vi "Editing VI Descriptions-2015.vi"() -> ()   [LabVIEW 2015]
doc: "Created IvanLis by LabVIEW Portal\nProfile: http://labviewportal.org/memberlist.php?mode=viewprofile&u=987\neMail: IvanLisanov@gMail.com\nTelegram: https://t.me/IvanLis"
panel:
  out "File Select":i32
  out "File Number":i32
  in  "DeSelect File":bool
  in  "DeSelect":bool
  in  "Select":bool
  in  "Change Description":bool
  in  "Get File List":bool
  out "Update":bool
  in  "File Type":T1(ring)
  in  "Folder Select":path
  in  "Description":string="Created IvanLis by LabVIEW Portal\nProfile: http://labviewportal.org/memberlist.php?mode=viewprofile&u=987\neMail: IvanLisanov@gMail.com\nTelegram: https://t.me/IvanLis"
  in  "Array of File":cluster{"Change":bool, "File":string}[](array[cluster])
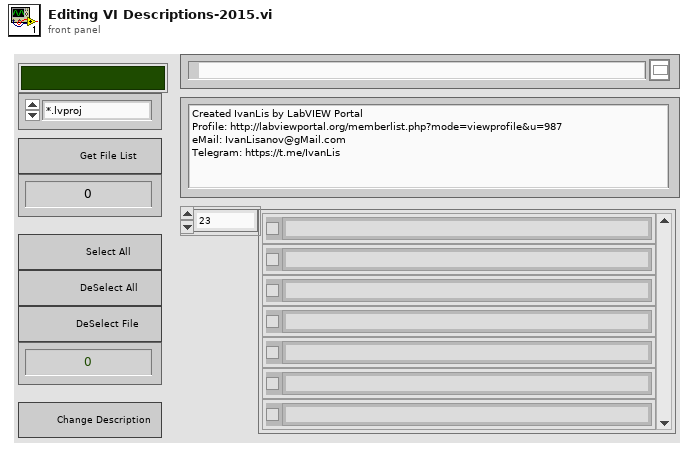
[diagram p1: front panel]
types:
  T1 = enum16{"*.lvproj", "*.vi", "*.ctl", "*.lvlib", "*.lvclass"}
  T2 = enum16{"open", "replace", "create", "open or create", "replace or create", "replace or create with confirmation"}
  T3 = typedef "LVRectTypeDef.ctl" = cluster{"Left":i16, "Top":i16, "Right":i16, "Bottom":i16}
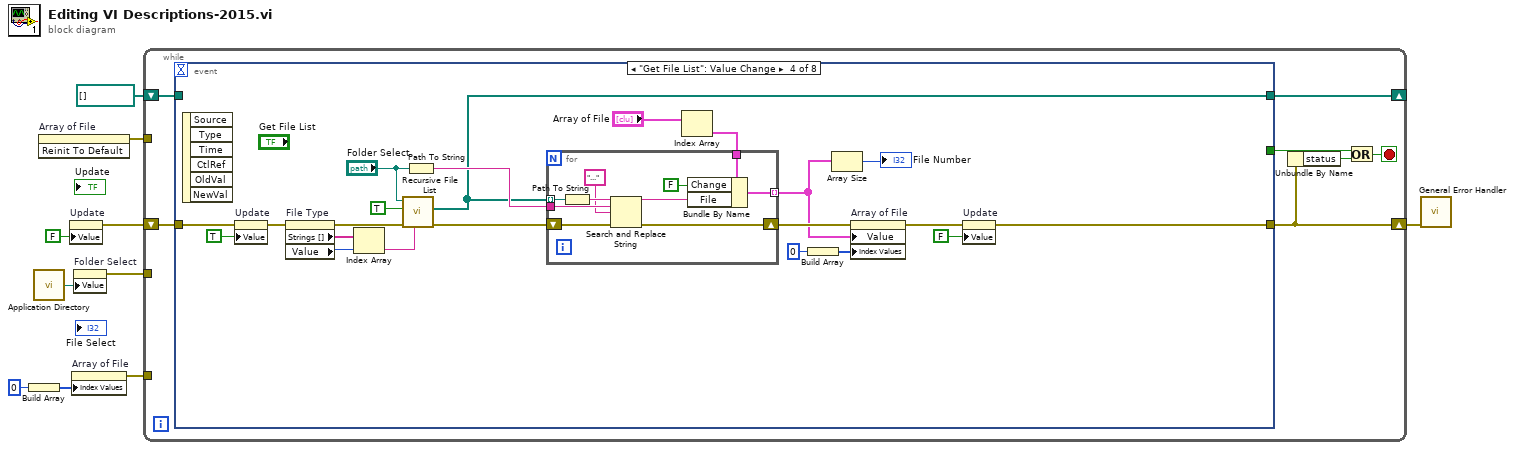
[diagram p0: block diagram]
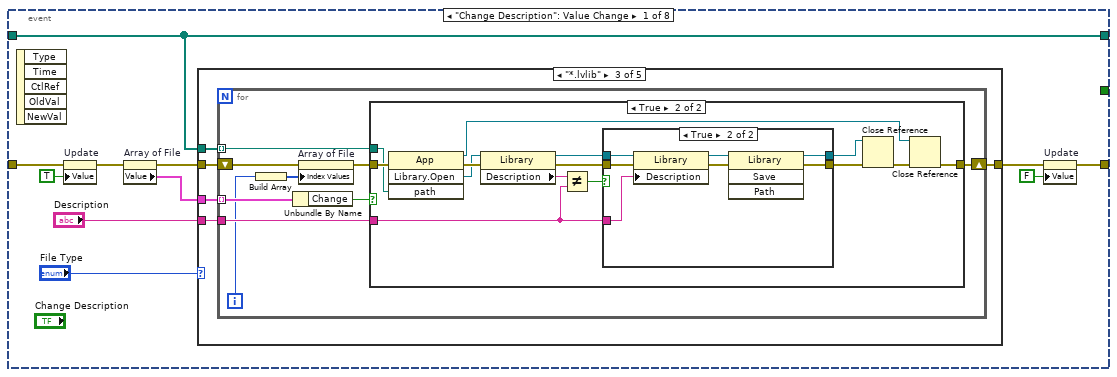
[diagram p2: hidden frame]
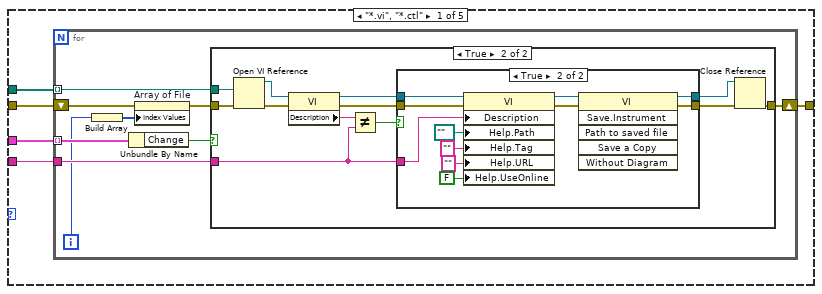
[diagram p3: hidden frame]
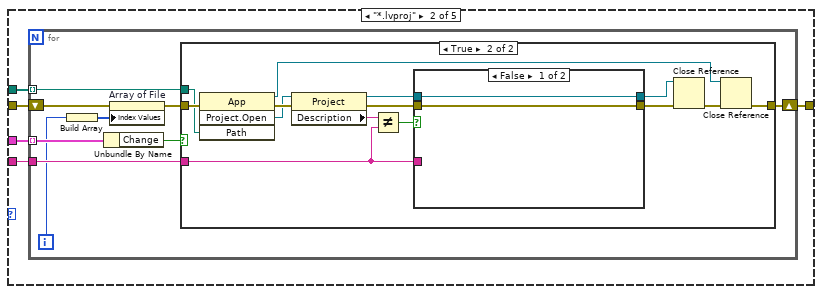
[diagram p6: hidden frame]
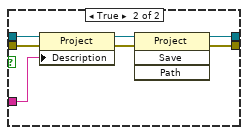
[diagram p8: hidden frame]
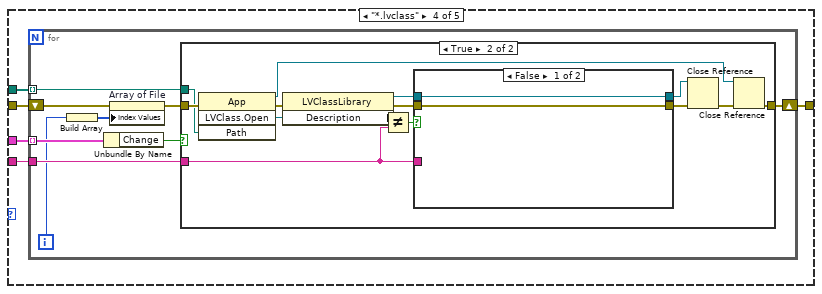
[diagram p11: hidden frame]
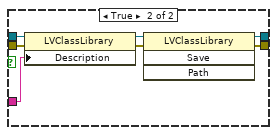
[diagram p13: hidden frame]
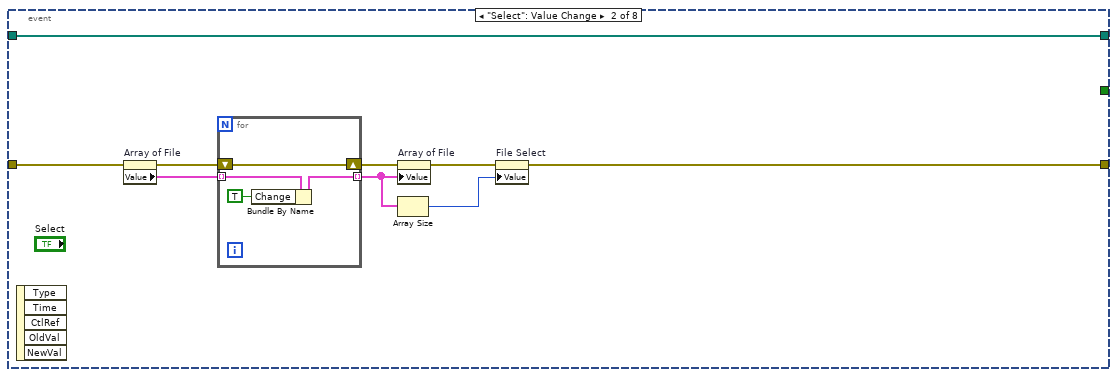
[diagram p15: hidden frame]
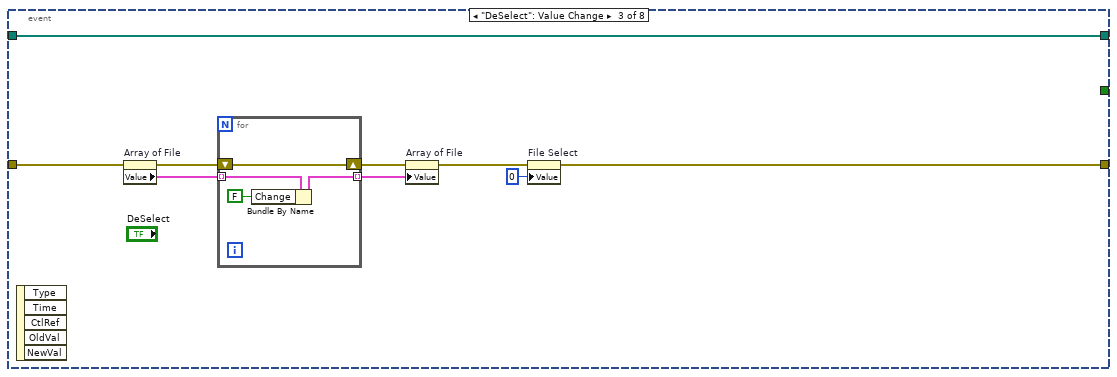
[diagram p16: hidden frame]
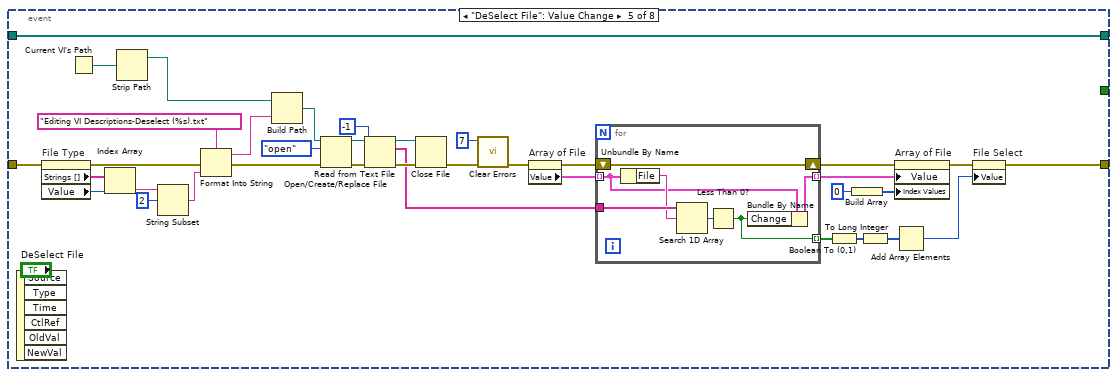
[diagram p17: hidden frame]
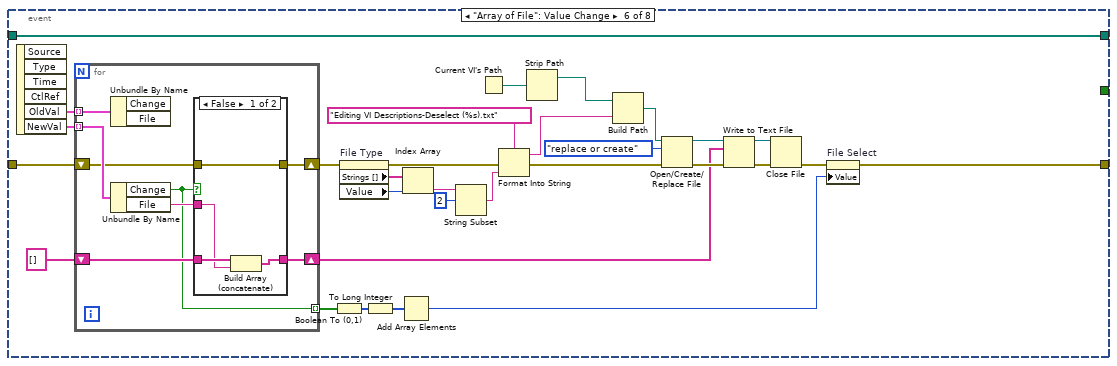
[diagram p18: hidden frame]
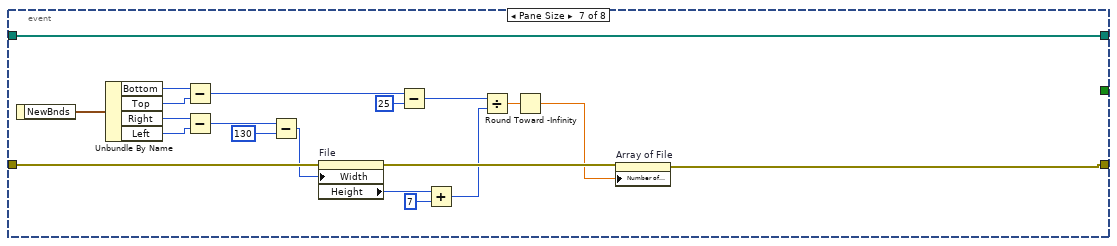
[diagram p20: hidden frame]
diagram:
  n1 = Build Array(u32 0) -> (w3:u32[])
  n2 = call <vilib>:"Application Directory.vi"() -> ("Application Directory"=w5:path)
  n3 = invoke on="Array of File" class="Arr (strict)" method="Reinit To Default"() -> (error out=w4:errorcluster)  [unwired: 3 in, 2 out]
  n4 = property on="Update" class="Bool (strict)"("Value"=FALSE ("Update")) -> (error out=w7:errorcluster)  [unwired: 2 in, 1 out]
  n5 = property on="Array of File" class="Arr (strict)"("Index Values"=w3) -> (error out=w1:errorcluster)  [unwired: 2 in, 1 out]
  n6 = property on="Folder Select" class="Path"("Value"=w5) -> (error out=w6:errorcluster)  [unwired: 2 in, 1 out]
  n7 = while {
    shift-right: [w16] -> w9
    shift-left: w7 -> [w17]
    shift-right: [w14] -> _
    shift-left: path[] [] ("All Files in Dir") -> [w13]
    tunnel: w6 -> [_]
    tunnel: w4 -> [_]
    tunnel: w1 -> [_]
    stop <- w15 stop-if-true
    n8 = event shown="[3] \"Get File List\": Value Change" {
      selector: _ -> [_ _ _ _ _ _ _ _]
      dyn-events: _ -> [_ _ _ _ _ _ _ _]
      timeout: _ -> [_ _ _ _ _ _ _ _]
      tunnel: w17 -> [w19 w192 w205 w213 w250 w312 w347 w351]
      tunnel: [w23 w186 w198 w220 w244 w289 w333 w351] -> w16
      tunnel: [w25 w189 w202 w224 w277 w311 w348 w350] -> w14
      tunnel: w13 -> [w25 w189 w202 _ w277 w311 w348 w350]
      tunnel: [_ _ _ _ _ _ _ w349] -> w12
      event "Change Description": Value Change {
        n9 = event-data() -> ()  [unwired: 1 in, 5 out]
        n10 = property on="Update" class="Bool (strict)"(error in=w19, "Value"=TRUE ("Update")) -> (error out=w20:errorcluster)  [unwired: 1 in, 1 out]
        n11 = property on="Array of File" class="Arr (strict)"(error in=w20) -> (error out=w27:errorcluster, "Value"=w26:cluster{"Change":bool, "File":string}[])  [unwired: 1 in, 1 out]
        n12 = case shown="\"*.lvlib\"" "File Type" {
          tunnel: "Description" -> [w33 w73 w111 w149 _]
          tunnel: w27 -> [w32 w72 w110 w148 w183]
          tunnel: w26 -> [w31 w71 w109 w147 _]
          tunnel: w25 -> [w30 w70 w108 w146 _]
          tunnel: [w29 w69 w107 w145 w183] -> w24
          frame "*.vi", "*.ctl" {
            n13 = for {
              tunnel: w33 -> [w41]
              shift-right: [w42] -> w29
              shift-left: w32 -> [w36]
              tunnel: w30 -> [w38] mode=indexing
              tunnel: w31 -> [w40] mode=indexing
              i -> [w34]
              n14 = Build Array(w34) -> (w37:i32[])
              n15 = Unbundle By Name(w40) -> ("Change"=w39:bool)
              n16 = property on="Array of File" class="Arr (strict)"(error in=w36, "Index Values"=w37) -> (error out=w35:errorcluster)  [unwired: 1 in, 1 out]
              n17 = case shown="True" w39 {
                tunnel: [w43 w55] -> w42
                tunnel: w41 -> [_ w46]
                tunnel: w35 -> [w43 w52]
                tunnel: w38 -> [_ w51]
                frame False {
                }
                frame True {
                  n18 = Open VI Reference(vi path=w51, error in (no error)=w52) -> (vi reference=w49:refnum<vi>, error out=w50:errorcluster)  [unwired: 4 in]
                  n19 = property class="VI"(reference=w49, error in=w50) -> (reference out=w48:refnum<vi>, error out=w44:errorcluster, "Description"=w47:string)
                  n20 = Not Equal?(x=w47, y=w46) -> (x != y?=w45:bool)
                  n21 = case shown="True" w45 {
                    tunnel: [w56 w66] -> w54
                    tunnel: [w57 w65] -> w53
                    tunnel: w48 -> [w57 w59]
                    tunnel: w46 -> [_ w58]
                    tunnel: w44 -> [w56 w60]
                    frame False {
                    }
                    frame True {
                      n22 = property class="VI"(reference=w59, error in=w60, "Description"=w58, "Help.Path"=path "" ("Help:Document Path"), "Help.Tag"="" ("Help:Document Tag"), "Help.URL"="" ("Help:Document Web URL"), "Help.UseOnline"=FALSE ("Help:Use Web URL")) -> (reference out=w67:refnum<vi>, error out=w68:errorcluster)
                      n23 = invoke class="VI" method="Save.Instrument"(reference=w67, error in=w68) -> (reference out=w65:refnum<vi>, error out=w66:errorcluster)  [unwired: 4 in, 4 out]
                    }
                  }
                  n24 = Close Reference(reference=w53, error in (no error)=w54) -> (error out=w55:errorcluster)
                }
              }
            }
          }
          frame "*.lvproj" {
            n25 = for {
              tunnel: w73 -> [w81]
              shift-right: [w82] -> w69
              shift-left: w72 -> [w76]
              tunnel: w70 -> [w78] mode=indexing
              tunnel: w71 -> [w80] mode=indexing
              i -> [w74]
              n26 = Build Array(w74) -> (w77:i32[])
              n27 = Unbundle By Name(w80) -> ("Change"=w79:bool)
              n28 = property on="Array of File" class="Arr (strict)"(error in=w76, "Index Values"=w77) -> (error out=w75:errorcluster)  [unwired: 1 in, 1 out]
              n29 = case shown="True" w79 {
                tunnel: [w83 w86] -> w82
                tunnel: w81 -> [_ w91]
                tunnel: w75 -> [w83 w95]
                tunnel: w78 -> [_ w87]
                frame False {
                }
                frame True {
                  n30 = invoke class="App" method="Project.Open"(error in=w95, "Path"=w87) -> (reference out=w84:refnum<vi>, error out=w94:errorcluster, "Project:Open"=w88:refnum<vi>)  [unwired: 2 in, 1 out]
                  n31 = property class="Project"(reference=w88, error in=w94) -> (reference out=w93:refnum<vi>, error out=w89:errorcluster, "Description"=w92:string)
                  n32 = Not Equal?(x=w92, y=w91) -> (x != y?=w90:bool)
                  n33 = case shown="False" w90 {
                    tunnel: [w98 w104] -> w97
                    tunnel: [w99 w103] -> w96
                    tunnel: w93 -> [w99 w101]
                    tunnel: w91 -> [_ w100]
                    tunnel: w89 -> [w98 w102]
                    frame False {
                    }
                    frame True {
                      n34 = property class="Project"(reference=w101, error in=w102, "Description"=w100) -> (reference out=w105:refnum<vi>, error out=w106:errorcluster)
                      n35 = invoke class="Project" method="Save"(reference=w105, error in=w106) -> (reference out=w103:refnum<vi>, error out=w104:errorcluster)  [unwired: 2 in, 2 out]
                    }
                  }
                  n36 = Close Reference(reference=w96, error in (no error)=w97) -> (error out=w85:errorcluster)
                  n37 = Close Reference(reference=w84, error in (no error)=w85) -> (error out=w86:errorcluster)
                }
              }
            }
          }
          frame "*.lvlib" {
            n38 = for {
              tunnel: w111 -> [w119]
              shift-right: [w120] -> w107
              shift-left: w110 -> [w114]
              tunnel: w108 -> [w116] mode=indexing
              tunnel: w109 -> [w118] mode=indexing
              i -> [w112]
              n39 = Build Array(w112) -> (w115:i32[])
              n40 = Unbundle By Name(w118) -> ("Change"=w117:bool)
              n41 = property on="Array of File" class="Arr (strict)"(error in=w114, "Index Values"=w115) -> (error out=w113:errorcluster)  [unwired: 1 in, 1 out]
              n42 = case shown="True" w117 {
                tunnel: [w121 w124] -> w120
                tunnel: w119 -> [_ w129]
                tunnel: w113 -> [w121 w133]
                tunnel: w116 -> [_ w125]
                frame False {
                }
                frame True {
                  n43 = invoke class="App" method="Library.Open"(error in=w133, "path"=w125) -> (reference out=w122:refnum<vi>, error out=w132:errorcluster, "Open Library"=w126:refnum<vi>)  [unwired: 2 in, 1 out]
                  n44 = property class="Library"(reference=w126, error in=w132) -> (reference out=w131:refnum<vi>, error out=w127:errorcluster, "Description"=w130:string)
                  n45 = Not Equal?(x=w130, y=w129) -> (x != y?=w128:bool)
                  n46 = case shown="True" w128 {
                    tunnel: [w136 w142] -> w135
                    tunnel: [w137 w141] -> w134
                    tunnel: w131 -> [w137 w139]
                    tunnel: w129 -> [_ w138]
                    tunnel: w127 -> [w136 w140]
                    frame False {
                    }
                    frame True {
                      n47 = property class="Library"(reference=w139, error in=w140, "Description"=w138) -> (reference out=w143:refnum<vi>, error out=w144:errorcluster)
                      n48 = invoke class="Library" method="Save"(reference=w143, error in=w144) -> (reference out=w141:refnum<vi>, error out=w142:errorcluster)  [unwired: 2 in, 2 out]
                    }
                  }
                  n49 = Close Reference(reference=w134, error in (no error)=w135) -> (error out=w123:errorcluster)
                  n50 = Close Reference(reference=w122, error in (no error)=w123) -> (error out=w124:errorcluster)
                }
              }
            }
          }
          frame "*.lvclass" {
            n51 = for {
              tunnel: w149 -> [w157]
              shift-right: [w158] -> w145
              shift-left: w148 -> [w152]
              tunnel: w146 -> [w154] mode=indexing
              tunnel: w147 -> [w156] mode=indexing
              i -> [w150]
              n52 = Build Array(w150) -> (w153:i32[])
              n53 = Unbundle By Name(w156) -> ("Change"=w155:bool)
              n54 = property on="Array of File" class="Arr (strict)"(error in=w152, "Index Values"=w153) -> (error out=w151:errorcluster)  [unwired: 1 in, 1 out]
              n55 = case shown="True" w155 {
                tunnel: [w159 w162] -> w158
                tunnel: w157 -> [_ w167]
                tunnel: w151 -> [w159 w171]
                tunnel: w154 -> [_ w163]
                frame False {
                }
                frame True {
                  n56 = invoke class="App" method="LVClass.Open"(error in=w171, "Path"=w163) -> (reference out=w160:refnum<vi>, error out=w170:errorcluster, "LVClass.Open"=w164:refnum<vi>)  [unwired: 2 in, 1 out]
                  n57 = property class="LVClassLibrary"(reference=w164, error in=w170) -> (reference out=w169:refnum<vi>, error out=w165:errorcluster, "Description"=w168:string)
                  n58 = Not Equal?(x=w168, y=w167) -> (x != y?=w166:bool)
                  n59 = case shown="False" w166 {
                    tunnel: [w174 w180] -> w173
                    tunnel: [w175 w179] -> w172
                    tunnel: w169 -> [w175 w177]
                    tunnel: w167 -> [_ w176]
                    tunnel: w165 -> [w174 w178]
                    frame False {
                    }
                    frame True {
                      n60 = property class="LVClassLibrary"(reference=w177, error in=w178, "Description"=w176) -> (reference out=w181:refnum<vi>, error out=w182:errorcluster)
                      n61 = invoke class="LVClassLibrary" method="Save"(reference=w181, error in=w182) -> (reference out=w179:refnum<vi>, error out=w180:errorcluster)  [unwired: 2 in, 2 out]
                    }
                  }
                  n62 = Close Reference(reference=w172, error in (no error)=w173) -> (error out=w161:errorcluster)
                  n63 = Close Reference(reference=w160, error in (no error)=w161) -> (error out=w162:errorcluster)
                }
              }
            }
          }
          frame Default {
          }
        }
        n64 = property on="Update" class="Bool (strict)"(error in=w24, "Value"=FALSE ("Update")) -> (error out=w23:errorcluster)  [unwired: 1 in, 1 out]
      }
      event "Select": Value Change {
        n65 = event-data() -> ()  [unwired: 1 in, 5 out]
        n66 = property on="Array of File" class="Arr (strict)"(error in=w192) -> (error out=w191:errorcluster, "Value"=w190:cluster{"Change":bool, "File":string}[])  [unwired: 1 in, 1 out]
        n67 = for {
          shift-right: [w194] -> w188
          shift-left: w191 -> [w194]
          tunnel: w190 -> [w196] mode=indexing
          tunnel: [w193] -> w185 mode=indexing
          n68 = Bundle By Name(cluster=w196, "Change"=TRUE) -> (w193:cluster{"Change":bool, "File":string})
        }
        n69 = property on="Array of File" class="Arr (strict)"(error in=w188, "Value"=w185) -> (error out=w187:errorcluster)  [unwired: 1 in, 1 out]
        n70 = Array Size(array=w185) -> (size(s)=w184:i32)
        n71 = property on="File Select" class="DigNum (strict)"(error in=w187, "Value"=w184) -> (error out=w186:errorcluster)  [unwired: 1 in, 1 out]
      }
      event "DeSelect": Value Change {
        n72 = event-data() -> ()  [unwired: 1 in, 5 out]
        n73 = property on="Array of File" class="Arr (strict)"(error in=w205) -> (error out=w204:errorcluster, "Value"=w203:cluster{"Change":bool, "File":string}[])  [unwired: 1 in, 1 out]
        n74 = for {
          shift-right: [w207] -> w201
          shift-left: w204 -> [w207]
          tunnel: w203 -> [w209] mode=indexing
          tunnel: [w206] -> w200 mode=indexing
          n75 = Bundle By Name(cluster=w209, "Change"=FALSE) -> (w206:cluster{"Change":bool, "File":string})
        }
        n76 = property on="Array of File" class="Arr (strict)"(error in=w201, "Value"=w200) -> (error out=w199:errorcluster)  [unwired: 1 in, 1 out]
        n77 = property on="File Select" class="DigNum (strict)"(error in=w199, "Value"=0 ("File Select")) -> (error out=w198:errorcluster)  [unwired: 1 in, 1 out]
      }
      event "Get File List": Value Change {
        n78 = event-data() -> ()  [unwired: 1 in, 6 out]
        n79 = property on="Update" class="Bool (strict)"(error in=w213, "Value"=TRUE ("Update")) -> (error out=w214:errorcluster)  [unwired: 1 in, 1 out]
        n80 = property on="File Type" class="Enum (strict)"(error in=w214) -> (error out=w223:errorcluster, "Strings []"=w222:string[], "Value"=w212:T1)  [unwired: 1 in, 1 out]
        n81 = Index Array(array=w222, index=w212) -> (element=w221:string)
        n82 = call <vilib>:"Recursive File List.vi"("pattern"=w221, "error in (no error)"=w223, "Treat LLBs as Folders?"=TRUE, "Folder Path"="Folder Select") -> ("error out"=w229:errorcluster, "All Files in Dir"=w224:path[])  [unwired: 3 in, 3 out]
        n83 = Path To String(path="Folder Select") -> (string=w227:string)
        n84 = Index Array(array="Array of File") -> (element=w231:cluster{"Change":bool, "File":string})  [unwired: 1 in]
        n85 = for {
          tunnel: w224 -> [w239] mode=indexing
          tunnel: w231 -> [w241]
          tunnel: w227 -> [w237]
          shift-right: [w233] -> w230
          shift-left: w229 -> [w234]
          tunnel: [w232] -> w210 mode=indexing
          n86 = Path To String(path=w239) -> (string=w238:string)
          n87 = Search and Replace String(input string=w238, search string=w237, replace string="..." ("replace string (\"\")"), error in=w234) -> (result string=w235:string, error out=w233:errorcluster)  [unwired: 4 in, 2 out]
          n88 = Bundle By Name(cluster=w241, "Change"=FALSE, "File"=w235) -> (w232:cluster{"Change":bool, "File":string})
        }
        n89 = Build Array(u32 0) -> (w216:u32[])
        n90 = Array Size(array=w210) -> (size(s)=→"File Number":i32)
        n91 = property on="Array of File" class="Arr (strict)"(error in=w230, "Value"=w210, "Index Values"=w216) -> (error out=w219:errorcluster)  [unwired: 1 in, 1 out]
        n92 = property on="Update" class="Bool (strict)"(error in=w219, "Value"=FALSE ("Update")) -> (error out=w220:errorcluster)  [unwired: 1 in, 1 out]
      }
      event "DeSelect File": Value Change {
        n93 = event-data() -> ()  [unwired: 1 in, 6 out]
        n94 = property on="File Type" class="Enum (strict)"(error in=w250) -> (error out=w254:errorcluster, "Strings []"=w256:string[], "Value"=w255:T1)  [unwired: 1 in, 1 out]
        n95 = Current VI's Path() -> (path=w274:path)
        n96 = Index Array(array=w256, index=w255) -> (element=w253:string)
        n97 = Strip Path(path=w274) -> (stripped path=w270:path)  [unwired: 1 out]
        n98 = String Subset(string=w253, offset (0)=2) -> (substring=w252:string)  [unwired: 1 in]
        n99 = Format Into String(format string="Editing VI Descriptions-Deselect (%s).txt" ("name or relative path"), error in=w254, w252) -> (resulting string=w248:string, error out=w249:errorcluster)  [unwired: 1 in]
        n100 = Build Path(base path=w270, name or relative path=w248) -> (appended path=w275:path)
        n101 = Open/Create/Replace File(file path (use dialog)=w275, error in=w249, operation (0:open)=T2."open") -> (refnum out=w273:refnum<file>, error out=w271:errorcluster)  [unwired: 3 in, 1 out]
        n102 = Read from Text File(file (use dialog)=w273, count=-1, error in=w271) -> (refnum out=w272:refnum<file>, text=w260:string[], error out=w269:errorcluster)  [unwired: 1 in, 1 out]
        n103 = Close File(refnum=w272, error in=w269) -> (error out=w263:errorcluster)  [unwired: 1 out]
        n104 = call <vilib>:"Clear Errors.vi"("error in (no error)"=w263, "specific error code to clear (0: all)"=7) -> ("error out"=w259:errorcluster)  [unwired: 4 in, 1 out]
        n105 = property on="Array of File" class="Arr (strict)"(error in=w259) -> (error out=w262:errorcluster, "Value"=w261:cluster{"Change":bool, "File":string}[])  [unwired: 1 in, 1 out]
        n106 = for {
          shift-right: [w281] -> w266
          shift-left: w262 -> [w281]
          tunnel: [w284] -> w267 mode=indexing
          tunnel: w261 -> [w280] mode=indexing
          tunnel: w260 -> [w283]
          tunnel: [w278] -> w247 mode=indexing
          n107 = Unbundle By Name(w280) -> ("File"=w282:string)
          n108 = Search 1D Array(1D array=w283, element=w282) -> (index of element=w279:i32)  [unwired: 1 in]
          n109 = Less Than 0?(x=w279) -> (x < 0?=w278:bool)
          n110 = Bundle By Name(cluster=w280, "Change"=w278) -> (w284:cluster{"Change":bool, "File":string})
        }
        n111 = Boolean To (0,1)(Boolean=w247) -> (0, 1=w246:i16[])
        n112 = Build Array(u32 0) -> (w264:u32[])
        n113 = To Long Integer(number=w246) -> (32bit integer=w242:i32[])
        n114 = property on="Array of File" class="Arr (strict)"(error in=w266, "Value"=w267, "Index Values"=w264) -> (error out=w245:errorcluster)  [unwired: 1 in, 1 out]
        n115 = Add Array Elements(numeric array=w242) -> (sum=w243:i32)
        n116 = property on="File Select" class="DigNum (strict)"(error in=w245, "Value"=w243) -> (error out=w244:errorcluster)  [unwired: 1 in, 1 out]
      }
      event "Array of File": Value Change {
        n117 = event-data() -> ("OldVal"=w314:cluster{"Change":bool, "File":string}[], "NewVal"=w313:cluster{"Change":bool, "File":string}[])  [unwired: 1 in, 4 out]
        n118 = for {
          tunnel: w314 -> [w322] mode=indexing
          tunnel: w313 -> [w321] mode=indexing
          shift-right: [w318] -> w296
          shift-left: w312 -> [w319]
          shift-right: [w316] -> w291
          shift-left: string[] [] -> [w320]
          tunnel: [w315] -> w286 mode=indexing
          n119 = Unbundle By Name(w322) -> ()  [unwired: 2 out]
          n120 = Unbundle By Name(w321) -> ("Change"=w315:bool, "File"=w317:string)
          n121 = case shown="False" w315 {
            tunnel: w319 -> [w326 w328]
            tunnel: [w326 w328] -> w318
            tunnel: w317 -> [w323 _]
            tunnel: w320 -> [w325 w327]
            tunnel: [w324 w327] -> w316
            frame False {
              n122 = Build Array (concatenate)(w325, w323) -> (w324:string[])
            }
            frame True {
            }
          }
        }
        n123 = Boolean To (0,1)(Boolean=w286) -> (0, 1=w288:i16[])
        n124 = property on="File Type" class="Enum (strict)"(error in=w296) -> (error out=w295:errorcluster, "Strings []"=w298:string[], "Value"=w297:T1)  [unwired: 1 in, 1 out]
        n125 = To Long Integer(number=w288) -> (32bit integer=w287:i32[])
        n126 = Add Array Elements(numeric array=w287) -> (sum=w285:i32)
        n127 = Index Array(array=w298, index=w297) -> (element=w294:string)
        n128 = String Subset(string=w294, offset (0)=2) -> (substring=w293:string)  [unwired: 1 in]
        n129 = Current VI's Path() -> (path=w307:path)
        n130 = Format Into String(format string="Editing VI Descriptions-Deselect (%s).txt" ("name or relative path"), error in=w295, w293) -> (resulting string=w299:string, error out=w301:errorcluster)  [unwired: 1 in]
        n131 = Strip Path(path=w307) -> (stripped path=w302:path)  [unwired: 1 out]
        n132 = Build Path(base path=w302, name or relative path=w299) -> (appended path=w308:path)
        n133 = Open/Create/Replace File(file path (use dialog)=w308, error in=w301, operation (0:open)=T2."replace or create") -> (refnum out=w306:refnum<file>, error out=w304:errorcluster)  [unwired: 3 in, 1 out]
        n134 = Write to Text File(file (use dialog)=w306, text=w291, error in=w304) -> (refnum out=w305:refnum<file>, error out=w303:errorcluster)  [unwired: 1 in, 1 out]
        n135 = Close File(refnum=w305, error in=w303) -> (error out=w290:errorcluster)  [unwired: 1 out]
        n136 = property on="File Select" class="DigNum (strict)"(error in=w290, "Value"=w285) -> (error out=w289:errorcluster)  [unwired: 1 in, 1 out]
      }
      event Pane Size {
        n137 = event-data() -> ("NewBnds"=w346:T3)  [unwired: 1 in]
        n138 = Unbundle By Name(w346) -> ("Bottom"=w340:i16, "Top"=w339:i16, "Right"=w345:i16, "Left"=w344:i16)
        n139 = Subtract(x=w340, y=w339) -> (x-y=w338:i16)
        n140 = Subtract(x=w345, y=w344) -> (x-y=w341:i16)
        n141 = Subtract(x=w341, y=i16 130) -> (x-y=w342:i16)
        n142 = property on="File" class="Str"(error in=w347, "Width"=w342) -> (error out=w334:errorcluster, "Height"=w330:u32)  [unwired: 1 in, 1 out]
        n143 = Subtract(x=w338, y=i16 25) -> (x-y=w336:i16)
        n144 = Add(x=w330, y=u32 7 ("y 2")) -> (x+y=w331:u32)
        n145 = Divide(x=w336, y=w331) -> (x/y=w335:dbl)
        n146 = Round Toward -Infinity(1:w335) -> (0:w332:dbl)
        n147 = property on="Array of File" class="Arr (strict)"(error in=w334, "Number of Rows"=w332) -> (error out=w333:errorcluster)  [unwired: 1 in, 1 out]
      }
      event Panel Close? {
        w349 = TRUE ("Discard?")
        n148 = event-data() -> ()  [unwired: 1 in, 4 out]
        n149 = event-data("Discard?"=w349) -> ()  [unwired: 1 in, 1 out]
      }
    }
    n150 = Unbundle By Name(w16) -> ("status"=w11:bool)
    n151 = Or(x=w12, y=w11) -> (x .or. y?=w15:bool)
  }
  n152 = call <vilib>:"General Error Handler.vi"("error in (no error)"=w9) -> ()  [unwired: 10 in, 5 out]
